vi "DataGraph_UpdateInterface.vi"(7 "Data In":T1={"FilePath"=path "", "Data State"=enum."Mass", "Data Plot Names"=["SelRange", "Data 1", "Data 2", "Data 3", "Data 4", "Data 5", "Data 6", "Data 7", "Data 8", "Data 9", "Data 10", "Data 11", "Data 12", "Data 13"], "DataArray"=[], "Volt Plot Names"=[], "VoltArray"=[], "UserDefine"={"Label"="", "Variant"=variant}, "Information"=variant}, 8 "error in (no error)":errorcluster, 9 "Info_Listbox":refnum<vi>, 10 "Title_Str":refnum<vi>, 11 "Mass_Graph":refnum<vi>) -> (0 "error out":errorcluster)   [LabVIEW 2018, in "DataGraphXControl.xctl"]
uses:
  DataGraphXControl.xctl
  DataGraph_Data.ctl
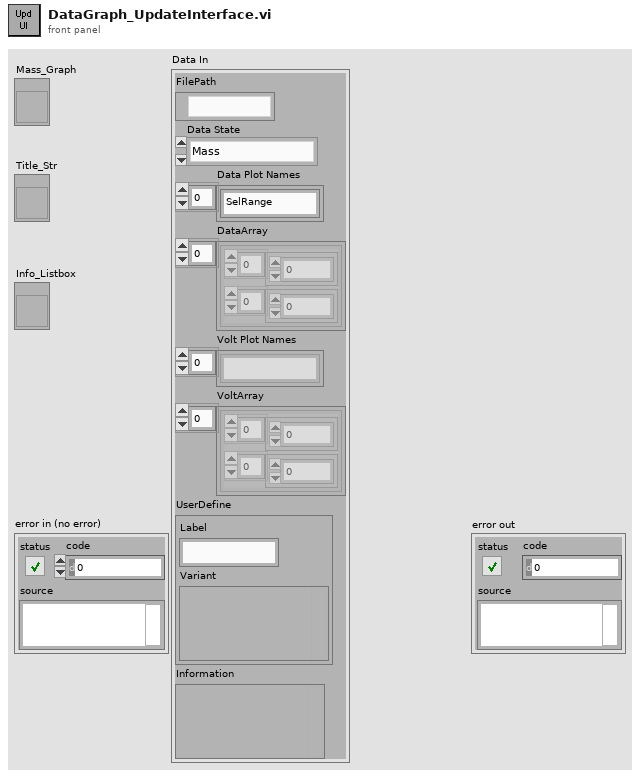
[diagram p1: front panel]
types:
  T1 = typedef "DataGraphXControl.xctl/DataGraph_Data.ctl" = cluster{"FilePath":path, "Data State":enum16{"Mass", "XIC"}, "Data Plot Names":string[], "DataArray":cluster{"X":dbl[], "Y":dbl[]}[], "Volt Plot Names":string[], "VoltArray":cluster{"X":dbl[], "Y":dbl[]}[], "UserDefine":cluster{"Label":string, "Variant":variant}, "Information":variant}
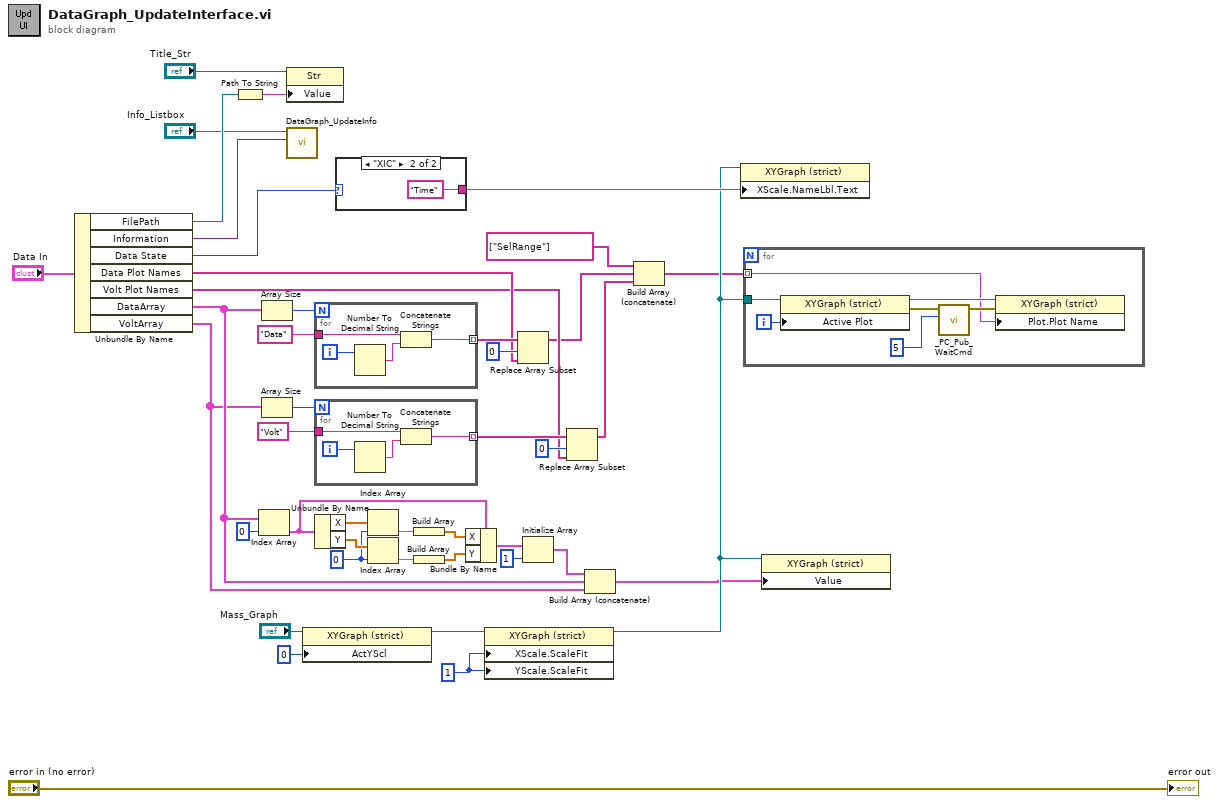
[diagram p0: block diagram]
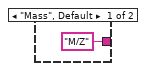
[diagram p2: hidden frame]
diagram:
  w29 = 0 ("index")
  w42 = u8 1 ("X Scale.Scale Fit")
  n1 = Unbundle By Name("Data In") -> ("FilePath"=w36:path, "Information"=w34:variant, "Data State"=w18:enum16{"Mass", "XIC"}, "Data Plot Names"=w9:string[], "Volt Plot Names"=w6:string[], "DataArray"=w19:cluster{"X":dbl[], "Y":dbl[]}[], "VoltArray"=w12:cluster{"X":dbl[], "Y":dbl[]}[])
  n2 = Path To String(path=w36) -> (string=w37:string)
  n3 = Index Array(array=w19, index=0) -> (element=w32:cluster{"X":dbl[], "Y":dbl[]})
  n4 = Array Size(array=w19) -> (size(s)=w16:i32)
  n5 = Array Size(array=w12) -> (size(s)=w14:i32)
  n6 = property class="Str"(reference="Title_Str", "Value"=w37) -> ()  [unwired: 1 in, 2 out]
  n7 = call "DataGraph_UpdateInfo.vi"("Information"=w34, "Info_Listbox"="Info_Listbox") -> ()  [unwired: 9 in, 1 out]
  n8 = property class="XYGraph (strict)"(reference="Mass_Graph", "ActYScl"=0 ("Active Y Scale")) -> (reference out=w1:refnum<vi>)  [unwired: 1 in, 1 out]
  n9 = for {
    N: w16 -> [_]
    tunnel: "Data" -> [w46]
    tunnel: [w44] -> w11 mode=indexing
    i -> [w47]
    n10 = Number To Decimal String(number=w47) -> (decimal integer string=w45:string)  [unwired: 1 in]
    n11 = Concatenate Strings(w46, w45) -> (w44:string)
  }
  n12 = for {
    N: w14 -> [_]
    tunnel: "Volt" -> [w50]
    tunnel: [w48] -> w7 mode=indexing
    i -> [w51]
    n13 = Number To Decimal String(number=w51) -> (decimal integer string=w49:string)  [unwired: 1 in]
    n14 = Concatenate Strings(w50, w49) -> (w48:string)
  }
  n15 = Unbundle By Name(w32) -> ("X"=w31:dbl[], "Y"=w30:dbl[])
  n16 = case shown="\"XIC\"" w18 {
    tunnel: ["M/Z" ("X Scale.Name Label.Text") "Time" ("X Scale.Name Label.Text")] -> w39
    frame "Mass", Default {
    }
    frame "XIC" {
    }
  }
  n17 = Index Array(array=w31, index=w29) -> (element=w28:dbl)
  n18 = Index Array(array=w30, index=w29) -> (element=w27:dbl)
  n19 = Build Array(w28) -> (w25:dbl[])
  n20 = Build Array(w27) -> (w26:dbl[])
  n21 = Bundle By Name(cluster=w32, "X"=w25, "Y"=w26) -> (w24:cluster{"X":dbl[], "Y":dbl[]})
  n22 = property class="XYGraph (strict)"(reference=w1, "XScale.ScaleFit"=w42, "YScale.ScaleFit"=w42) -> (reference out=w38:refnum<vi>)  [unwired: 1 in, 1 out]
  n23 = Replace Array Subset(array=w11, new element=w9, index=0) -> (w5:string[])
  n24 = Initialize Array(w24, 1 ("dimension size")) -> (w20:cluster{"X":dbl[], "Y":dbl[]}[])
  n25 = Replace Array Subset(array=w7, new element=w6, index=0) -> (w4:string[])
  n26 = Build Array (concatenate)(w20, w19, w12) -> (w23:cluster{"X":dbl[], "Y":dbl[]}[])
  n27 = Build Array (concatenate)(string[] ["SelRange"] ("array"), w5, w4) -> (w22:string[])
  n28 = property class="XYGraph (strict)"(reference=w38, "XScale.NameLbl.Text"=w39) -> ()  [unwired: 1 in, 2 out]
  n29 = for {
    tunnel: w22 -> [w54] mode=indexing
    tunnel: w38 -> [w60]
    i -> [w58]
    n30 = property class="XYGraph (strict)"(reference=w60, "Active Plot"=w58) -> (reference out=w56:refnum<vi>, error out=w59:errorcluster)  [unwired: 1 in]
    n31 = call "_PC_Pub_WaitCmd.vi"("milliseconds to wait"=u32 5, "error in (no error)"=w59) -> ("error out"=w55:errorcluster)  [unwired: 9 in]
    n32 = property class="XYGraph (strict)"(reference=w56, error in=w55, "Plot.Plot Name"=w54) -> ()  [unwired: 2 out]
  }
  n33 = property class="XYGraph (strict)"(reference=w38, "Value"=w23) -> ()  [unwired: 1 in, 2 out]
  "error out" <- "error in (no error)"
